vi "Action.vi"(8 "error in (no error)":errorcluster, 10 "Actor in":refnum<class "Tamagotchi Basic Actor.lvclass">, 11 "Fixed Bug Message in":refnum<class "Fixed Bug Message.lvclass">) -> (0 "error out":errorcluster, 2 "Actor out":refnum<class "Tamagotchi Basic Actor.lvclass">, 3 "Fixed Bug Message out":refnum<class "Fixed Bug Message.lvclass">)   [LabVIEW 2026, in "Fixed Bug Message.lvclass"]
uses:
  Fixed Bug Message.lvclass
  Tamagotchi Basic Actor/Tamagotchi Basic Actor.lvclass
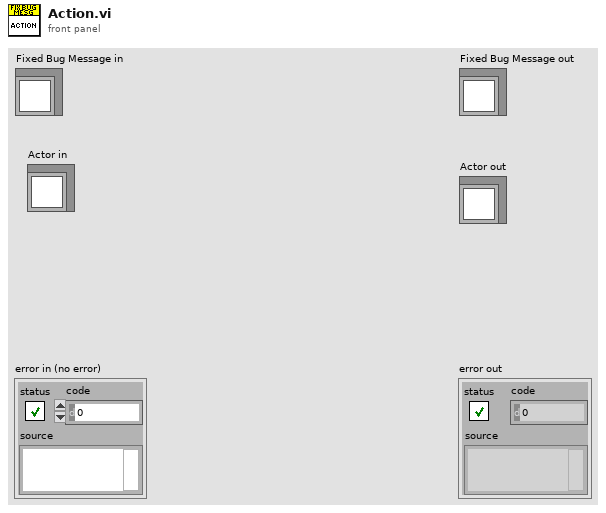
[diagram p1: front panel]
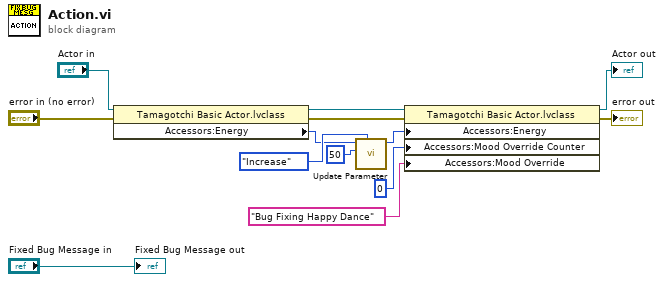
[diagram p0: block diagram]
diagram:
  n1 = property class="Tamagotchi Basic Actor.lvclass"(reference="Actor in", error in="error in (no error)") -> (reference out=w4:refnum<class "Tamagotchi Basic Actor.lvclass">, error out=w3:errorcluster, "Accessors:Energy"=w9:i16)
  n2 = call "Update Parameter.vi"("Action"=enum16{"Increase", "Decrease"}."Increase", "Modifier"=i16 50 ("y"), "Parameter"=w9) -> ("New Value"=w6:i16)  [unwired: 8 in]
  n3 = property class="Tamagotchi Basic Actor.lvclass"(reference=w4, error in=w3, "Accessors:Energy"=w6, "Accessors:Mood Override Counter"=u32 0 ("Mood Override Counter"), "Accessors:Mood Override"="Bug Fixing Happy Dance" ("Mood Override")) -> (reference out=→"Actor out":refnum<class "Tamagotchi Basic Actor.lvclass">, error out=→"error out":errorcluster)
  "Fixed Bug Message out" <- "Fixed Bug Message in"
